vi "Calculate_Non-zero_Displac-s_in_Matrix-1.vi"(1 "[IN] Displacements \nFrm-to-Frm In Cols":dbl[][](array[numeric])) -> (0 "[OUT] Number of \n(X,Y,dX,dY) displ-s":i32)   [LabVIEW 2013]
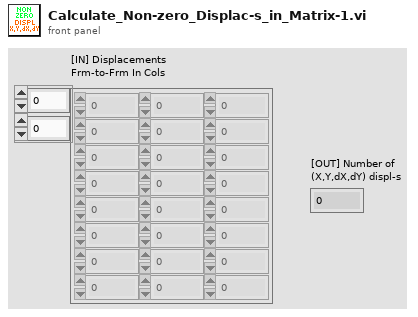
[diagram p1: front panel]
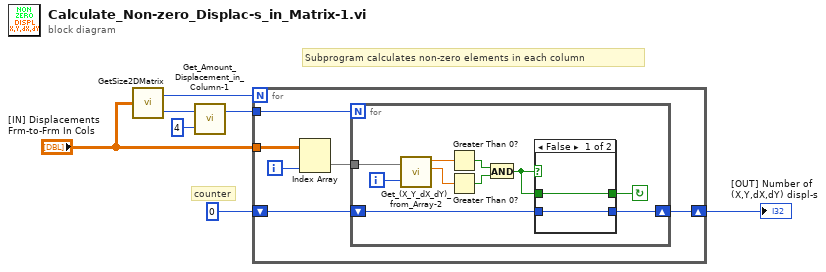
[diagram p0: block diagram]
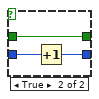
[diagram p2: hidden frame]
diagram:
  # "Subprogram calculates non-zero elements in each column"
  # "counter"
  n1 = call "GetSize2DMatrix.vi"("Array IN (2D)"="[IN] Displacements \nFrm-to-Frm In Cols") -> ("# Cols"=w7:i32, "# Rows"=w4:i32)
  n2 = call "Get_Amount_Displacement_in_Column-1.vi"("multiplier"=4, "# Rows"=w4) -> ("Displ amount"=w2:i32)  [unwired: 1 out]
  n3 = for {
    N: w7 -> [_]
    shift-right: [w8] -> w1
    shift-left: 0 -> [w9]
    tunnel: "[IN] Displacements \nFrm-to-Frm In Cols" -> [w13]
    tunnel: w2 -> [w11]
    i -> [w12]
    n4 = Index Array(array=w13, index (col)=w12) -> (element=w10:dbl[])  [unwired: 1 in]
    n5 = for {
      N: w11 -> [_]
      tunnel: w10 -> [w23]
      shift-right: [w14] -> w8
      shift-left: w9 -> [w15]
      i -> [w22]
      stop <- w16 continue-if-true
      n6 = call "Get_(X_Y_dX_dY)_from_Array-2.vi"("(X,Y,dX,dY)"=w23, "Index of Displacement"=w22) -> ("X"=w21:dbl, "Y"=w20:dbl)  [unwired: 2 out]
      n7 = Greater Than 0?(x=w21) -> (x > 0?=w19:bool)
      n8 = Greater Than 0?(x=w20) -> (x > 0?=w18:bool)
      n9 = And(x=w19, y=w18) -> (x .and. y?=w17:bool)
      n10 = case shown="False" w17 {
        tunnel: w17 -> [w25 w28]
        tunnel: [w25 w28] -> w16
        tunnel: w15 -> [w24 w27]
        tunnel: [w24 w26] -> w14
        frame False {
        }
        frame True {
          n11 = Increment(x=w27) -> (x+1=w26:i32)
        }
      }
    }
  }
  "[OUT] Number of \n(X,Y,dX,dY) displ-s" <- w1
